vi "[SubVI]KpKd_Scale.vi"(3 "Hip Angle":dbl) -> (0 "Scaled Kd":dbl, 1 "Scaled Kp":dbl)   [LabVIEW 2018]
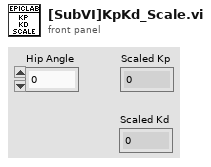
[diagram p1: front panel]
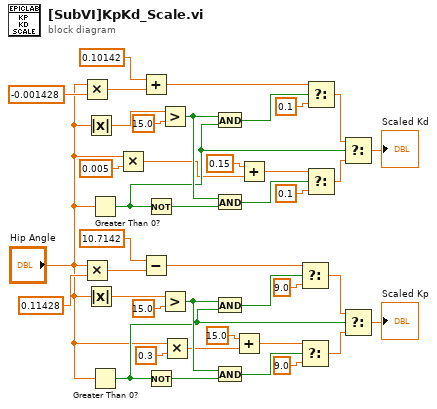
[diagram p0: block diagram]
diagram:
  n1 = Multiply(x="Hip Angle", y=-0.001428) -> (x*y=w6:dbl)
  n2 = Multiply(x="Hip Angle", y=0.11428) -> (x*y=w25:dbl)
  n3 = Absolute Value(x="Hip Angle") -> (abs(x)=w14:dbl)
  n4 = Absolute Value(x="Hip Angle") -> (abs(x)=w34:dbl)
  n5 = Greater Than 0?(x="Hip Angle") -> (x > 0?=w15:bool)
  n6 = Greater Than 0?(x="Hip Angle") -> (x > 0?=w35:bool)
  n7 = Multiply(x="Hip Angle", y=0.005) -> (x*y=w11:dbl)
  n8 = Add(x=0.10142 ("y"), y=w6) -> (x+y=w5:dbl)
  n9 = Subtract(x=10.7142 ("y"), y=w25) -> (x-y=w24:dbl)
  n10 = Not(x=w15) -> (.not. x?=w17:bool)
  n11 = Not(x=w35) -> (.not. x?=w37:bool)
  n12 = Greater?(x=w14, y=15.0) -> (0:w16:bool)
  n13 = Greater?(x=w34, y=15.0) -> (0:w36:bool)
  n14 = Multiply(x="Hip Angle", y=0.3) -> (x*y=w31:dbl)
  n15 = And(x=w16, y=w15) -> (x .and. y?=w4:bool)
  n16 = And(x=w16, y=w17) -> (x .and. y?=w18:bool)
  n17 = And(x=w36, y=w35) -> (x .and. y?=w23:bool)
  n18 = And(x=w36, y=w37) -> (x .and. y?=w38:bool)
  n19 = Add(x=15.0 ("y"), y=w31) -> (x+y=w40:dbl)
  n20 = Add(x=0.15 ("y"), y=w11) -> (x+y=w20:dbl)
  n21 = Select(t=w24, s=w23, f=9.0) -> (s? t:f=w28:dbl)
  n22 = Select(t=w40, s=w38, f=9.0) -> (s? t:f=w39:dbl)
  n23 = Select(t=w5, s=w4, f=0.1) -> (s? t:f=w9:dbl)
  n24 = Select(t=w20, s=w18, f=0.1) -> (s? t:f=w19:dbl)
  n25 = Select(t=w9, s=w15, f=w19) -> (s? t:f=→"Scaled Kd":dbl)
  n26 = Select(t=w28, s=w35, f=w39) -> (s? t:f=→"Scaled Kp":dbl)
